vi "Update Plot Legends.vi"(8 "error in (no error)":errorcluster, 11 "HistorianCharting in":refnum<class "HistorianCharting.lvclass">) -> (0 "error out":errorcluster, 3 "HistorianCharting out":refnum<class "HistorianCharting.lvclass">)   [LabVIEW 2020, in "VolatusGUIElements.lvlib" / "HistorianCharting.lvclass"]
uses:
  HistorianCharting.lvclass
  HistorianCharting.lvclass/HistorianCharting.ctl
  VolatusGUI/Historian Charting Manager/Scale.ctl
  Volatus/VolatusAPI/VolatusAPI.lvclass/VolatusAPI.ctl
  lv-vecto/Vecto/Channel DBL/Channel DBL.lvclass/Channel DBL.ctl
  lv-vecto/Vecto/ChannelService/Lookup Double Channel.vi
  lv-vecto/Vecto/Group DBL/Value by Index.vi
  VolatusGUI/Historian Charting Manager/Historian Charting Manager.lvclass
  lv-vecto/Vecto/Channel DBL/Channel DBL.lvclass
  Volatus/VolatusAPI/VolatusAPI.lvclass
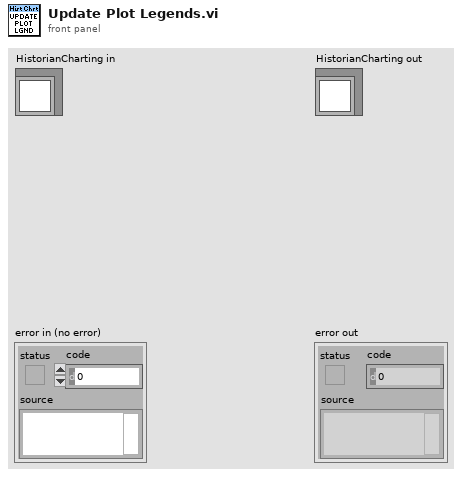
[diagram p1: front panel]
types:
  T1 = typedef "VolatusGUI.lvlib/Historian Charting Manager.lvclass/Plot Config.ctl" = cluster{"Channel":string, "Visible":bool, "Color":u32, "Scale":T2}
  T2 = typedef "VolatusGUI.lvlib/Historian Charting Manager.lvclass/Scale.ctl" = enum16{"Left", "Right"}
  T3 = cluster{"Channel":string, "Value":dbl, "Color":u32, "Scale":bool, "Visible":bool}
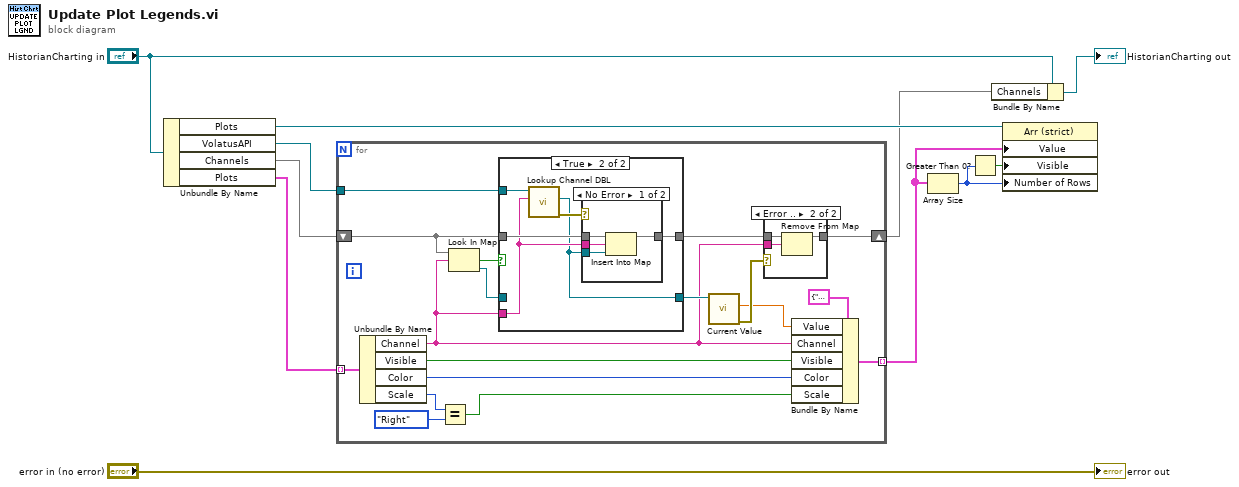
[diagram p0: block diagram]
diagram:
  n1 = Unbundle By Name("HistorianCharting in") -> ("Plots"=w8:refnum<vi>, "VolatusAPI"=w6:refnum<class "VolatusAPI.lvclass">, "Channels"=w7:map{string, refnum<class "Channel DBL.lvclass">}, "Plots"=w9:T1[])
  n2 = for {
    tunnel: w9 -> [w28] mode=indexing
    tunnel: [w21] -> w3 mode=indexing
    shift-right: [w13] -> w4
    shift-left: w7 -> [w16]
    tunnel: w6 -> [w15]
    n3 = Unbundle By Name(w28) -> ("Channel"=w12:string, "Visible"=w26:bool, "Color"=w25:u32, "Scale"=w24:T2)
    n4 = Equal?(x=w24, y=Scale."Right") -> (x = y?=w22:bool)
    n5 = Look In Map(map=w16, key=w12) -> (key not found?=w20:bool, value=w19:refnum<class "Channel DBL.lvclass">)  [unwired: 1 in]
    n6 = case shown="True" w20 {
      tunnel: w19 -> [w35 _]
      tunnel: [w35 w37] -> w18
      tunnel: w16 -> [w34 w39]
      tunnel: w12 -> [_ w38]
      tunnel: w15 -> [_ w40]
      tunnel: [w34 w36] -> w14
      frame False {
      }
      frame True {
        n7 = call "Lookup Channel DBL.vi"("Name"=w38, "VolatusAPI in"=w40) -> ("error out"=w41:errorcluster, "Channel DBL"=w37:refnum<class "Channel DBL.lvclass">)  [unwired: 7 in, 1 out]
        n8 = case shown="No Error" w41 {
          tunnel: w39 -> [w45 w46]
          tunnel: w38 -> [w44 _]
          tunnel: w37 -> [w43 _]
          tunnel: [w42 w46] -> w36
          frame No Error {
            n9 = Insert Into Map(map in=w45, key=w44, value=w43) -> (map out=w42:map{string, refnum<class "Channel DBL.lvclass">})  [unwired: 2 out]
          }
          frame Error {
          }
        }
      }
    }
    n10 = call "Current Value.vi"("Channel in"=w18) -> ("error out"=w29:errorcluster, "Scaled"=w17:dbl)  [unwired: 6 in, 3 out]
    n11 = case shown="Error .." w29 {
      tunnel: w14 -> [w30 w33]
      tunnel: [w30 w32] -> w13
      tunnel: w12 -> [_ w31]
      frame No Error {
      }
      frame Error {
        n12 = Remove From Map(10:w31, 11:w33) -> (3:w32:map{string, refnum<class "Channel DBL.lvclass">})  [unwired: 2 out]
      }
    }
    n13 = Bundle By Name(cluster=T3 {"Channel"="", "Value"=0.0, "Color"=16777215, "Scale"=FALSE, "Visible"=FALSE} ("Plot"), "Value"=w17, "Channel"=w12, "Visible"=w26, "Color"=w25, "Scale"=w22) -> (w21:T3)
  }
  n14 = Array Size(array=w3) -> (size(s)=w2:i32)
  n15 = Greater Than 0?(x=w2) -> (x > 0?=w1:bool)
  n16 = Bundle By Name(cluster="HistorianCharting in", "Channels"=w4) -> (→"HistorianCharting out":refnum<class "HistorianCharting.lvclass">)
  n17 = property class="Arr (strict)"(reference=w8, "Value"=w3, "Visible"=w1, "Number of Rows"=w2) -> ()  [unwired: 1 in, 2 out]
  "error out" <- "error in (no error)"
